vi "dB_to_K.vi"(1 "Усиление (дБ)":dbl) -> (0 "Коэффициент усиления":dbl)   [LabVIEW 2025]
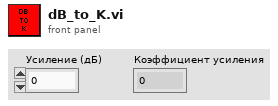
[diagram p1: front panel]
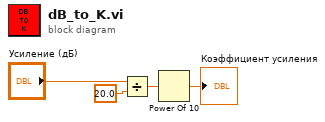
[diagram p0: block diagram]
diagram:
  n1 = Divide(x="Усиление (дБ)", y=20.0) -> (x/y=w2:dbl)
  n2 = Power Of 10(x=w2) -> (10^x=→"Коэффициент усиления":dbl)
